vi "HXG2_CoilDataFGV.vi"(7 "FGVctrl":enum16{"Write", "Pass"}(ring), 8 "error in (no error)":errorcluster, 11 "String Data":string[](array[string])) -> (0 "error out":errorcluster, 2 "Header":string[](array[string]), 5 "Data Out":string[](array[string]))   [LabVIEW 2012]
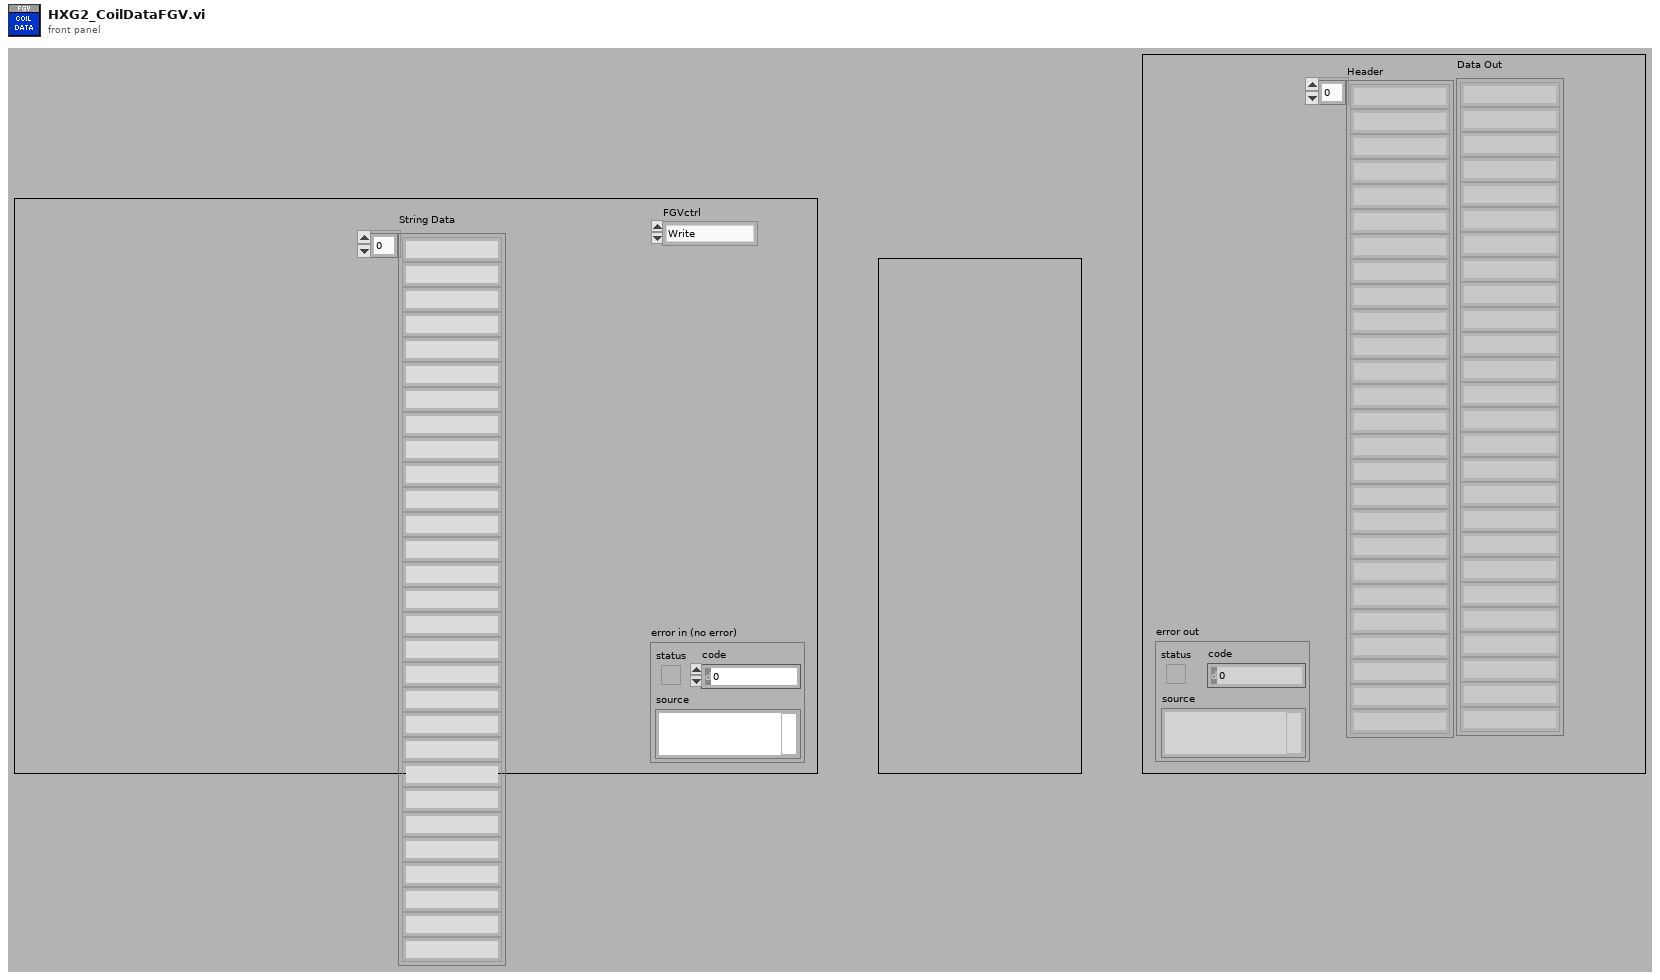
[diagram p1: front panel]
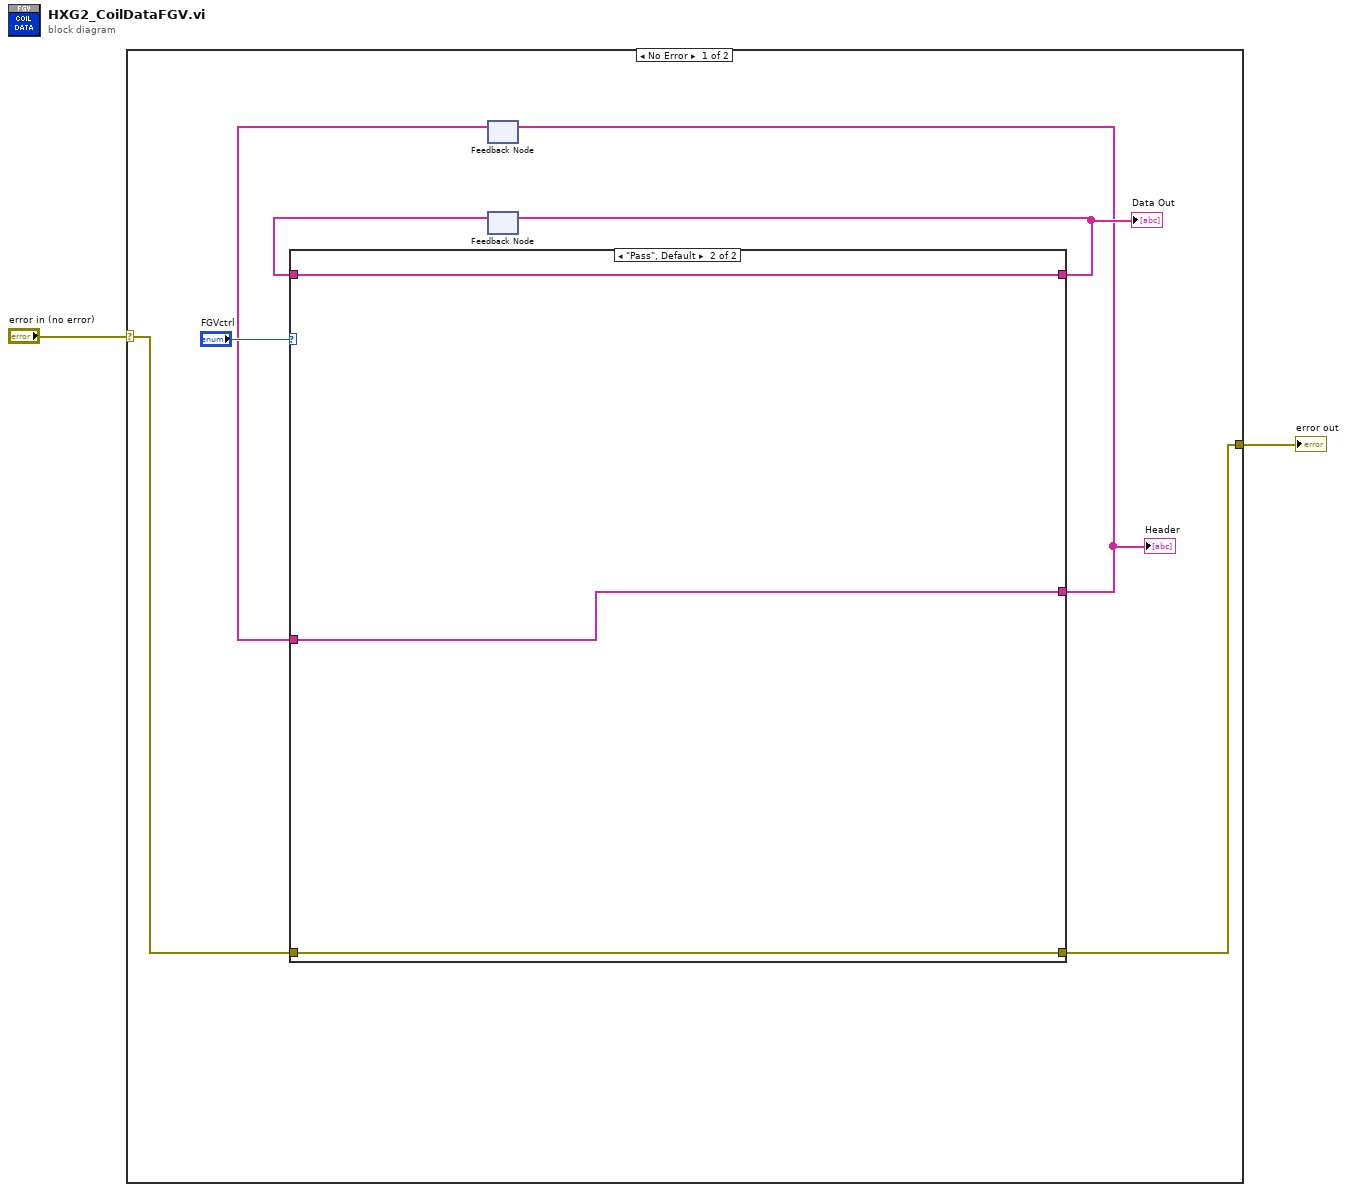
[diagram p0: block diagram]
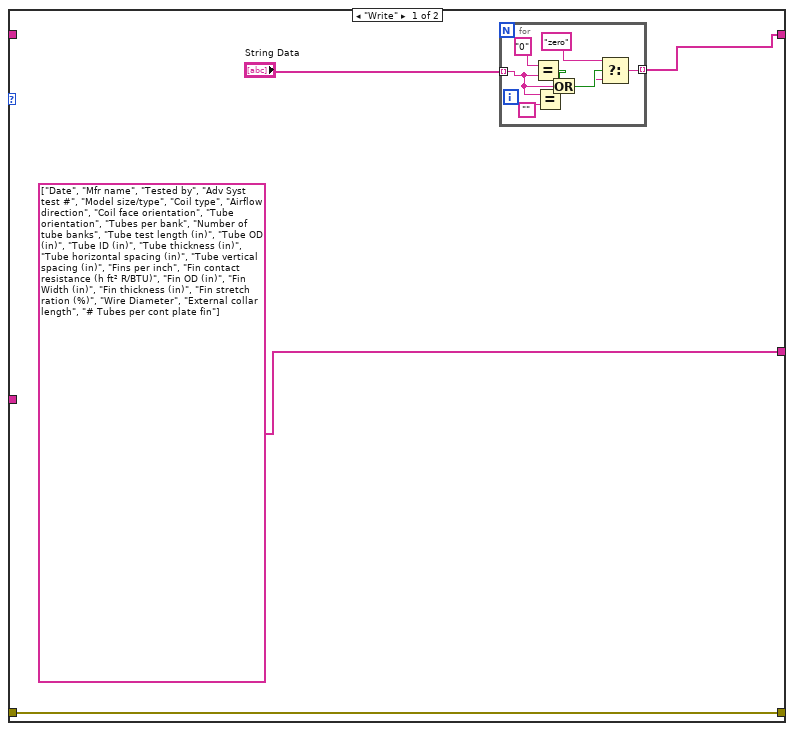
[diagram p2: hidden frame]
diagram:
  n1 = case shown="No Error" "error in (no error)" {
    selector: "error in (no error)" -> [w8 w25]
    tunnel: [w7 w25] -> w2
    frame No Error {
      n2 = feedback #1() -> (w4:string[])  [unwired: 1 in]
      n3 = feedback #2() -> (w5:string[])  [unwired: 1 in]
      n4 = case shown="\"Pass\", Default" "FGVctrl" {
        tunnel: w8 -> [w13 w24]
        tunnel: [w13 w24] -> w7
        tunnel: [w12 w23] -> w6
        tunnel: w5 -> [_ w23]
        tunnel: [string[] ["Date", "Mfr name", "Tested by", "Adv Syst test #", "Model size/type", "Coil type", "Airflow direction", "Coil face orientation", "Tube orientation", "Tubes per bank", "Number of tube banks", "Tube test length (in)", "Tube OD (in)", "Tube ID (in)", "Tube thickness (in)", "Tube horizontal spacing (in)", "Tube vertical spacing (in)", "Fins per inch", "Fin contact resistance (h ft² R/BTU)", "Fin OD (in)", "Fin Width (in)", "Fin thickness (in)", "Fin stretch ration (%)", "Wire Diameter", "External collar length", "# Tubes per cont plate fin"] ("Header") w22] -> w3
        tunnel: w4 -> [_ w22]
        frame "Write" {
          n5 = for {
            tunnel: "String Data" -> [w14] mode=indexing
            tunnel: [w19] -> w12 mode=indexing
            n6 = Equal?(x="0", y=w14) -> (x = y?=w17:bool)
            n7 = Equal?(x=w14, y="") -> (x = y?=w16:bool)
            n8 = Or(x=w17, y=w16) -> (x .or. y?=w15:bool)
            n9 = Select(t="zero" ("x"), s=w15, f=w14) -> (s? t:f=w19:string)
          }
        }
        frame "Pass", Default {
        }
      }
      "Data Out" <- w6
      "Header" <- w3
      n10 = feedback-in #1(w3) -> ()
      n11 = feedback-in #2(w6) -> ()
    }
    frame Error {
    }
  }
  "error out" <- w2
